vi "Update Status Message for Test.vi"(11 "Example Parallel Test in":refnum<class "Example Parallel Test.lvclass">) -> ()   [LabVIEW 2015, in "Example Parallel Test.lvclass"]
uses:
  Example Parallel Test.lvclass
  Test Class/Test Class.lvclass
  Classes/Application/Class/Application.lvclass
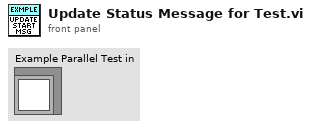
[diagram p1: front panel]
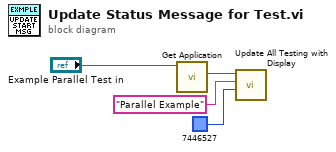
[diagram p0: block diagram]
diagram:
  n1 = call "Get Application.vi"("Test Class in"="Example Parallel Test in") -> ("Application.lvlib:Application.lvclass"=w2:refnum<class "Application.lvclass">)  [unwired: 9 in, 1 out]
  n2 = call "Update All Testing with Display.vi"("BG Color"=u32 7446527, "Message ('')"="Parallel Example", "Application in"=w2) -> ()  [unwired: 7 in, 2 out]
